vi "MicroPulse TCP read header + count.vi"(8 "error in (no error)":errorcluster, 9 "TCP timeout":i32, 11 "connection ID":refnum<k5>) -> (0 "error out":errorcluster, 1 "TCP timeout":i32, 2 "bytes to read":i32, 3 "connection ID out":refnum<k5>, 4 "total msg length":i32, 5 "hdr (+count)":string, 7 "Header Byte":u8 format="%.0x")   [LabVIEW 2026, in "MicroPulse_Driver.lvlib"]
uses:
  MicroPulse_Driver.lvlib
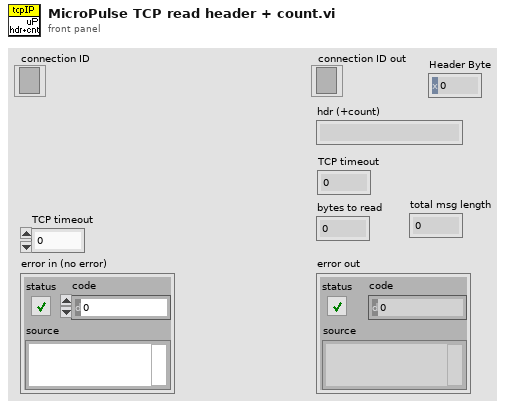
[diagram p1: front panel]
types:
  T1 = cluster{"fixed hdr":u8[], "fixed count":i32[], "variable hdr":u8[], "variable count":i32[]}
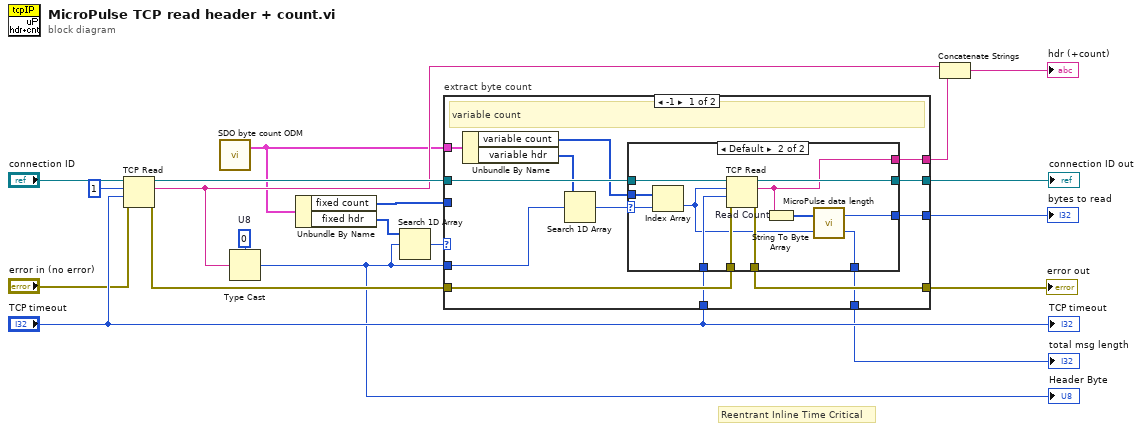
[diagram p0: block diagram]
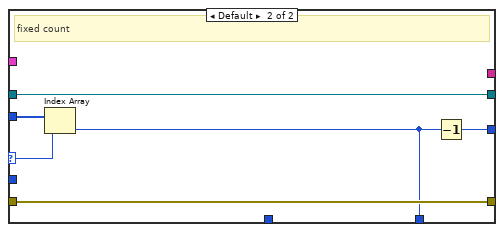
[diagram p3: hidden frame]
diagram:
  w2 = u8 0  # U8
  # "Reentrant Inline Time Critical"
  n1 = TCP Read(connection ID="connection ID", bytes to read=1, error in (no error)="error in (no error)", 9:"TCP timeout") -> (connection ID out=w17:refnum<k5>, data out=w8:string, error out=w13:errorcluster)  [unwired: 1 out]
  n2 = call "SDO byte count ODM.vi"() -> ("byte counts"=w3:T1)  [unwired: 5 in]
  n3 = Type Cast(type=w2, x=w8) -> (*(type *) &x=w1:u8)
  "Header Byte" <- w1
  n4 = Unbundle By Name(w3) -> ("fixed count"=w4:i32[], "fixed hdr"=w5:u8[])
  n5 = Search 1D Array(1D array=w5, element=w1) -> (index of element=w7:i32)  [unwired: 1 in]
  n6 = case "extract byte count" shown="-1" w7 {
    selector: w7 -> [_ w52]
    tunnel: [w21 w48] -> w9
    tunnel: w4 -> [_ w51]
    tunnel: w13 -> [w32 w49]
    tunnel: w17 -> [w31 w50]
    tunnel: [w30 w50] -> w16
    tunnel: [w29 _] -> w6
    tunnel: [w28 w49] -> w15
    tunnel: w1 -> [w26 _]
    tunnel: w3 -> [w24 _]
    tunnel: "TCP timeout" -> [w22 _]
    tunnel: [w20 w47] -> w11
    frame -1 {
      # "variable count"
      n7 = Unbundle By Name(w24) -> ("variable count"=w25:i32[], "variable hdr"=w27:u8[])
      n8 = Search 1D Array(1D array=w27, element=w26) -> (index of element=w23:i32)  [unwired: 1 in]
      n9 = case shown="Default" w23 {
        selector: w23 -> [_ w38]
        tunnel: [_ w35] -> w21
        tunnel: w32 -> [w34 w45]
        tunnel: w31 -> [w33 w44]
        tunnel: [w33 w43] -> w30
        tunnel: [_ w42] -> w29
        tunnel: [w34 w41] -> w28
        tunnel: w25 -> [_ w40]
        tunnel: w22 -> [_ w39]
        tunnel: [_ w36] -> w20
        frame -1 {
        }
        frame Default {
          n10 = Index Array(array=w40, index=w38) -> (element=w37:i32)
          n11 = TCP Read "Read Count"(connection ID=w44, bytes to read=w37, error in (no error)=w45, 9:w39) -> (connection ID out=w43:refnum<k5>, data out=w42:string, error out=w41:errorcluster)  [unwired: 1 out]
          n12 = String To Byte Array(string=w42) -> (unsigned byte array=w46:u8[])
          n13 = call "MicroPulse data length.vi"("count length"=w37, "[U8] count bytes"=w46) -> ("total msg length"=w36:i32, "data length"=w35:i32)
        }
      }
    }
    frame Default {
      # "fixed count"
      n14 = Index Array(array=w51, index=w52) -> (element=w47:i32)
      n15 = Decrement(x=w47) -> (x-1=w48:i32)
    }
  }
  "bytes to read" <- w9
  "error out" <- w15
  "connection ID out" <- w16
  "total msg length" <- w11
  n16 = Concatenate Strings(w8, w6) -> (→"hdr (+count)":string)
  "TCP timeout" <- "TCP timeout"
